vi "Position Updated.vi"(8 "error in (no error)":errorcluster, 10 "New Position":dbl, 11 "Business Logic in":refnum<class "Business Logic.lvclass">) -> (0 "error out":errorcluster, 3 "Business Logic out":refnum<class "Business Logic.lvclass">)   [LabVIEW 2025, in "Business Logic.lvlib" / "Business Logic.lvclass"]
uses:
  Business Logic.lvclass
  Business Logic.lvclass/Business Logic.ctl
  User Interface Messages/Update Current Position Msg/Update Current Position Msg.lvclass
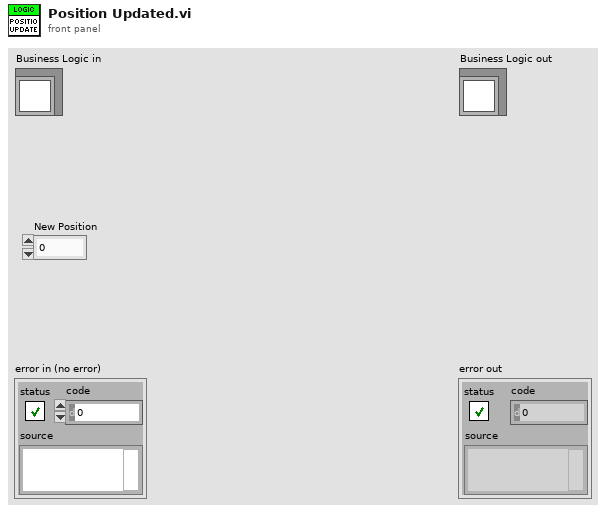
[diagram p1: front panel]
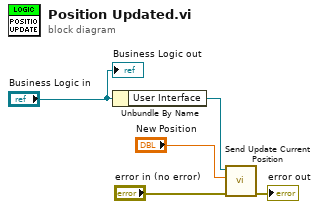
[diagram p0: block diagram]
diagram:
  n1 = Unbundle By Name("Business Logic in") -> ("User Interface"=w4:refnum<class "Message Enqueuer.lvclass">)
  n2 = call "Send Update Current Position.vi"("error in (no error)"="error in (no error)", "Current Position"="New Position", "Message Enqueuer"=w4) -> ("error out"=→"error out":errorcluster)  [unwired: 7 in, 1 out]
  "Business Logic out" <- "Business Logic in"
